vi "libssh2_sftp_opendir.vi"(8 "error in (no error)":errorcluster, 10 "path":string, 11 "sftp":T2) -> (0 "error out":errorcluster, 3 "sftp handle":T1)   [LabVIEW 2013, in "libssh2.lvlib"]
doc: "Open directory handle for reading on SFTP."
uses:
  libssh2.lvlib
  SFTP Refnum.ctl
  SFTP Handle Refnum.ctl
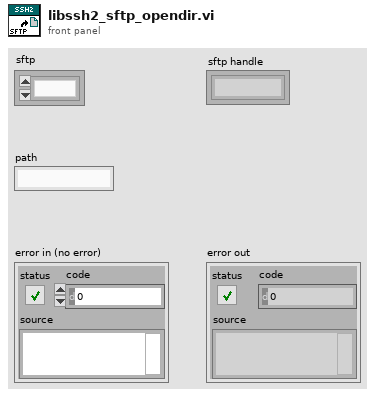
[diagram p1: front panel]
types:
  T1 = typedef "libssh2.lvlib/SFTP Handle Refnum.ctl" = refnum<k1>
  T2 = typedef "libssh2.lvlib/SFTP Refnum.ctl" = refnum<k1>
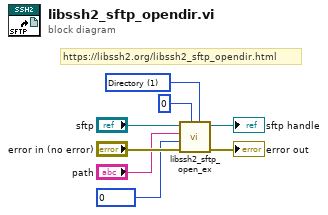
[diagram p0: block diagram]
diagram:
  w1 = u32 0 items=["LIBSSH2_FXF_READ"=1, "LIBSSH2_FXF_WRITE"=2, "LIBSSH2_FXF_APPEND"=4, "LIBSSH2_FXF_CREAT"=8, "LIBSSH2_FXF_TRUNC"=16, "LIBSSH2_FXF_EXCL"=32] ("flags")
  w2 = 1 items=["File", "Directory"] ("open_type (0 = file)")
  # "https://libssh2.org/libssh2_sftp_opendir.html"
  n1 = call "libssh2_sftp_open_ex.vi"("open_type (0 = file)"=w2, "mode"=0, "error in (no error)"="error in (no error)", "flags"=w1, "filename"="path", "sftp"="sftp") -> ("error out"=→"error out":errorcluster, "sftp handle"=→"sftp handle":T1)  [unwired: 4 in]
